vi "EditorPDF setPDFMainGraph.vi"(8 "error in (no error)":errorcluster, 11 "CreatePDF in":refnum<class "CreatePDF.lvclass">) -> (0 "error out":errorcluster, 3 "CreatePDF out":refnum<class "CreatePDF.lvclass">)   [LabVIEW 2018, in "CreatePDF.lvclass"]
uses:
  CreatePDF.lvclass
  CreatePDF.lvclass/CreatePDF.ctl
  Sub/EditorSub createPictureMain.vi
  <vilib>/Simplicity AI/SAI_PDF_API/Classes/Context/Methods/Public/Low Level/Add/SAI_PDF_Add Line Feed.vi
  <vilib>/Simplicity AI/SAI_PDF_API/Classes/Context/Context.lvclass
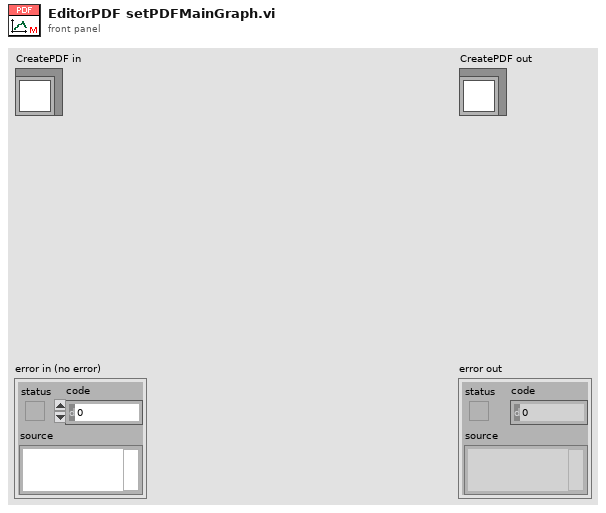
[diagram p1: front panel]
types:
  T1 = typedef "imagedata.ctl" = cluster{"image type":i32, "image depth":i32, "image":u8[], "mask":u8[], "colors":u32[], "Rectangle":cluster{"left":i16, "top":i16, "right":i16, "bottom":i16}}
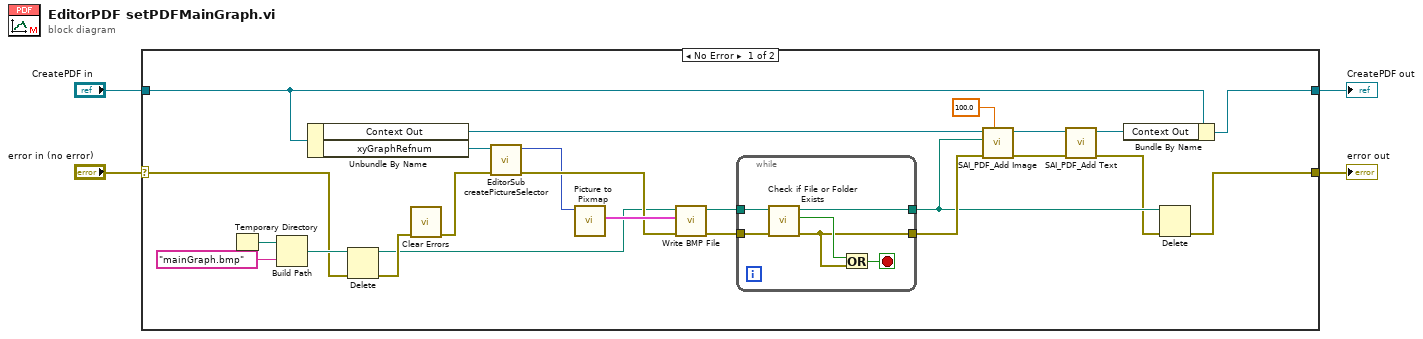
[diagram p0: block diagram]
diagram:
  n1 = case shown="No Error" "error in (no error)" {
    selector: "error in (no error)" -> [w10 w36]
    tunnel: [w17 w36] -> w3
    tunnel: [w27 w35] -> w1
    tunnel: "CreatePDF in" -> [w28 w35]
    frame No Error {
      n2 = Temporary Directory() -> (w25:path)
      n3 = Build Path(base path=w25, name or relative path="mainGraph.bmp") -> (appended path=w13:path)
      n4 = Unbundle By Name(w28) -> ("Context Out"=w18:refnum<class "Context.lvclass">, "xyGraphRefnum"=w16:refnum<vi>)
      n5 = Delete(path (use dialog)=w13, error in=w10) -> (deleted path=w11:path, error out=w12:errorcluster)  [unwired: 4 out]
      n6 = call <vilib>:"Clear Errors.vi"("error in (no error)"=w12) -> ("error out"=w9:errorcluster)  [unwired: 5 in, 1 out]
      n7 = call-poly "EditorSub createPictureSelector.vi"("error in (no error)"=w9, "XY Graph"=w16) -> ("error out"=w15:errorcluster, "2D Picture"=w14:picture)  [unwired: 8 in]
      n8 = call <vilib>:"Picture to Pixmap.vi"("picture"=w14) -> ("image data"=w26:T1)  [unwired: 9 in, 1 out]
      n9 = call <vilib>:"Write BMP File.vi"("error in (no error)"=w15, "image data"=w26, "path to BMP file"=w11) -> ("error out"=w21:errorcluster, "path"=w22:path)  [unwired: 7 in]
      n10 = while {
        tunnel: w22 -> [w34]
        tunnel: w21 -> [w33]
        tunnel: [w30] -> w20
        tunnel: [w29] -> w19
        stop <- w31 stop-if-true
        n11 = call <vilib>:"Check if File or Folder Exists.vi"("error in (no error)"=w33, "path"=w34) -> ("error out"=w30:errorcluster, "file or folder exists?"=w32:bool, "dup path"=w29:path)  [unwired: 7 in]
        n12 = Or(x=w32, y=w30) -> (x .or. y?=w31:bool)
      }
      n13 = call <vilib>:"SAI_PDF_Add Image.vi"("Scale Percentage (100%)"=sgl 100.0, "error in"=w20, "File Name"=w19, "Context In"=w18) -> ("error out"=w7:errorcluster, "Context Out"=w8:refnum<class "Context.lvclass">)  [unwired: 2 in, 4 out]
      n14 = call-poly <vilib>:"SAI_PDF_Add Text.vi"("error in"=w7, "Context In"=w8) -> ("error out"=w6:errorcluster, "Context Out"=w5:refnum<class "Context.lvclass">)  [unwired: 2 in, 6 out]
      n15 = Bundle By Name(cluster=w28, "Context Out"=w5) -> (w27:refnum<class "CreatePDF.lvclass">)
      n16 = Delete(path (use dialog)=w19, error in=w6) -> (error out=w17:errorcluster)  [unwired: 5 out]
    }
    frame Error {
    }
  }
  "error out" <- w3
  "CreatePDF out" <- w1
